vi "Set Position AE.vi"() -> (0 "Cursor Y":dbl)   [LabVIEW 2014]
uses:
  FPGA-7842R-Reference.ctl
panel:
  in  "Set Position":bool
  out "Channel 1":sgl[][](graph)
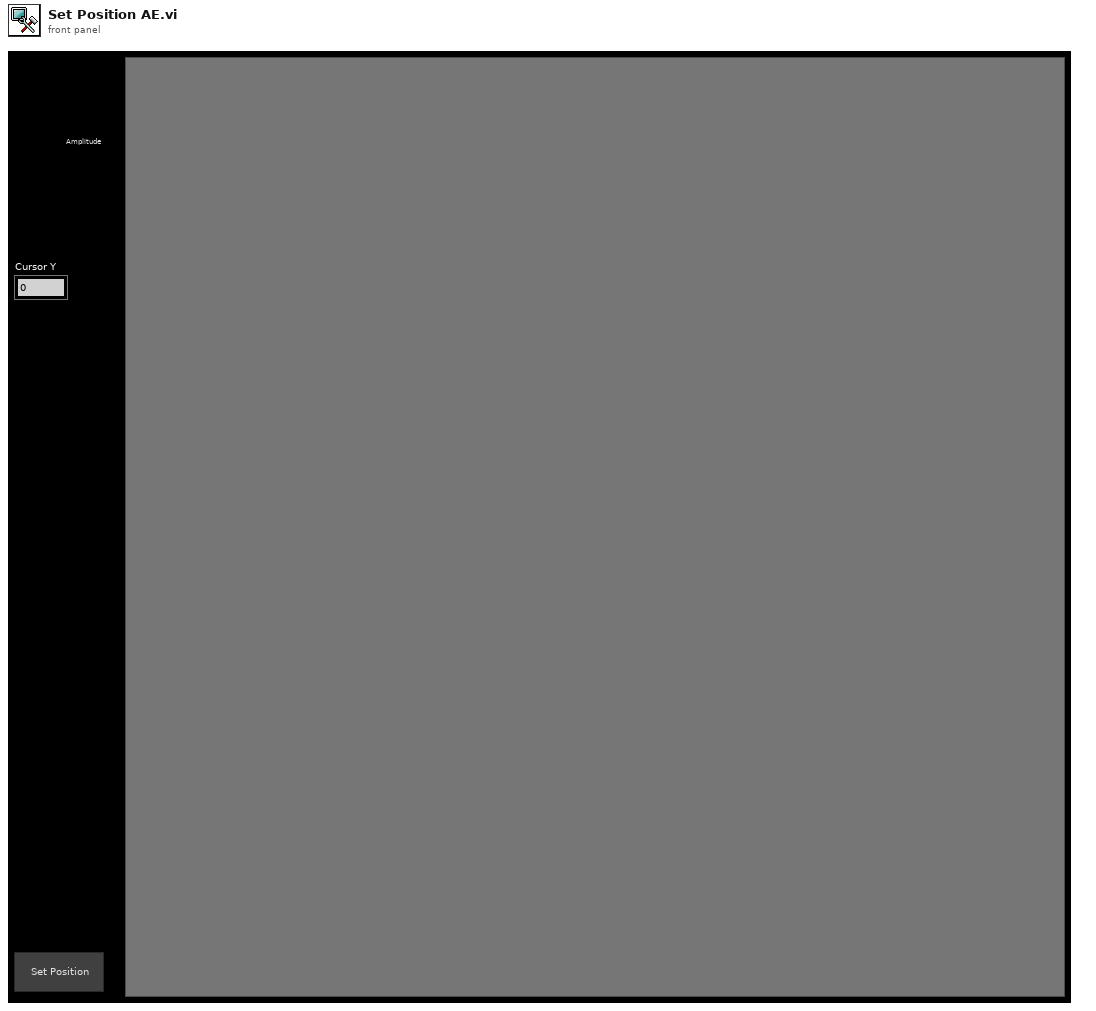
[diagram p1: front panel]
types:
  T1 = typedef "FPGA-7842R-Reference.ctl" = enum16{"Stage Control", "Laser Control", "Unused Axis I16", "Exit", "Set Res Mirror", "Set Galvo", "Current Frame for Capture", "Default", "Close FPGA", "Stop Waveforms", "Start Waveforms", "Shutter Control", "Initialize"}
  T2 = typedef "Image Acquisition Parameters.ctl" = cluster{"Scan Type":enum16{"Sample Scanning", "Beam Scanning"}, "Scan Mode":enum16{"XY", "XZ", "YZ", "XYZ"}, "Fast Axis Frequency (Hz)":dbl, "Image Format":u16, "Line Accumulations":u16, "Frames Per Capture":u16, "Frames Accumulations":u16, "Image Dimension (um)":dbl[], "Number of Z Steps":u16, "Z Steps Size (um)":dbl, "Pixel Size (nm)":dbl[], "Customized Image Format":dbl[]}
  T3 = typedef "Manual Controls V2.ctl" = cluster{"Galvo 1 Position (I16)":i16, "Galvo 2 Position (I16)":i16, "X Axis Voltage (I16)":i16, "Y Axis Voltage (I16)":i16, "Z Axis Voltage (I16)":i16, "Res Mirror Amp (I16)":i16, "Res Mirror Mute":bool, "Upper Shutter":bool, "Lower Shutter":bool}
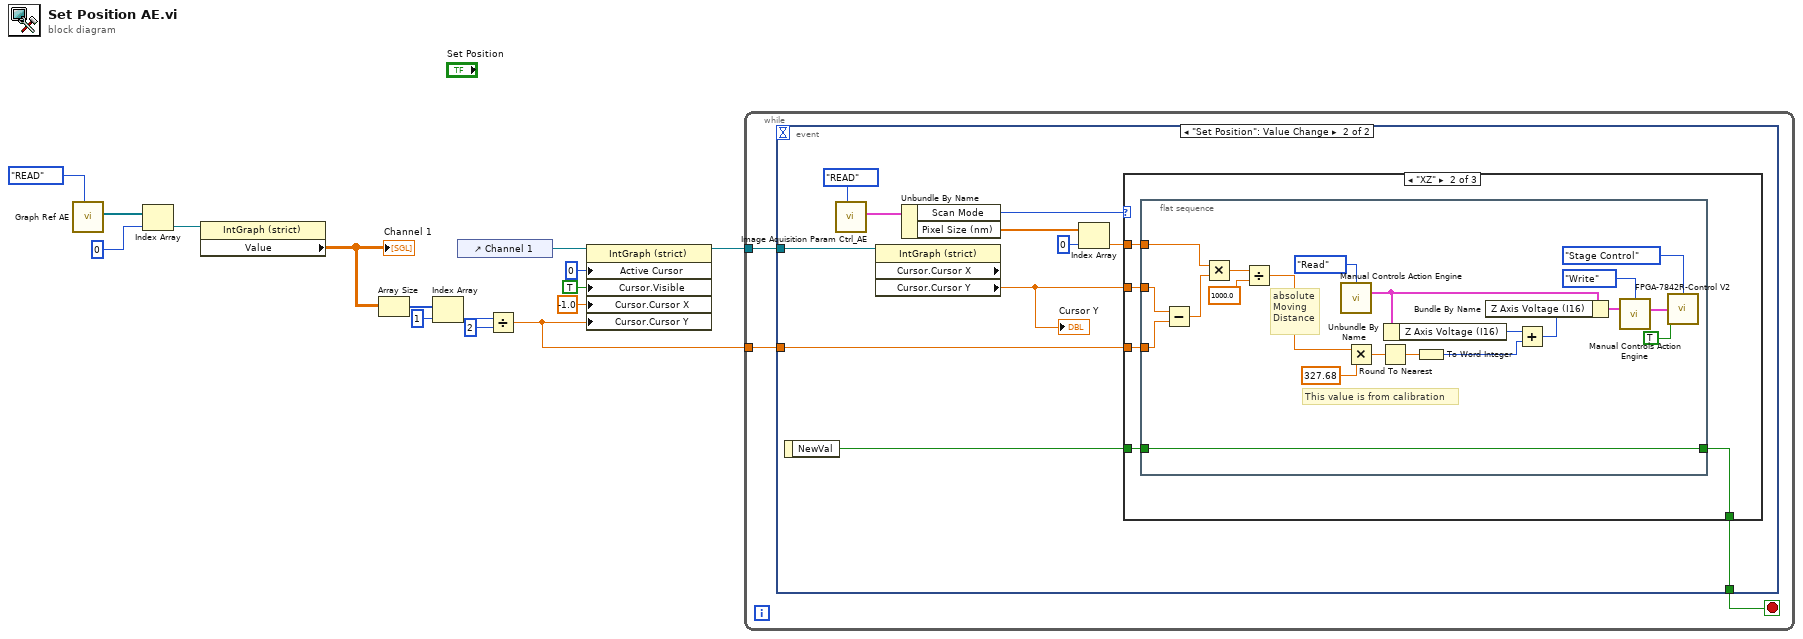
[diagram p0: block diagram]
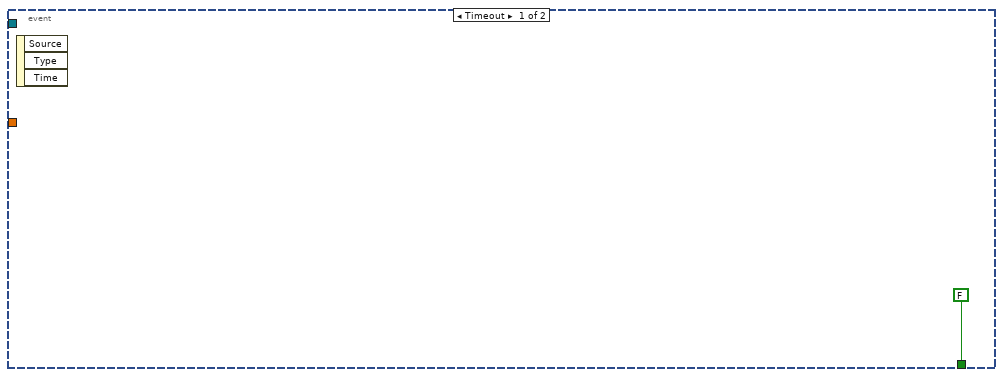
[diagram p2: hidden frame]
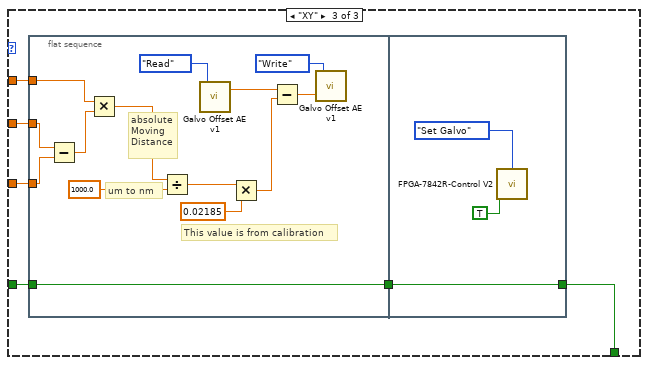
[diagram p4: hidden frame]
diagram:
  n1 = call "Graph Ref AE.vi"("Action"=enum16{"READ", "WRITE"}."READ") -> ("Graph Ref Out"=w11:refnum<vi>[])  [unwired: 10 in]
  n2 = Index Array(array=w11, index=0) -> (element=w9:refnum<vi>)
  n3 = property class="IntGraph (strict)"(reference=w9) -> ("Value"=w4:sgl[][])  [unwired: 1 in, 2 out]
  "Channel 1" <- w4
  n4 = Array Size(array=w4) -> (size(s)=w8:i32[])
  n5 = Index Array(array=w8, index=1) -> (element=w6:i32)
  n6 = control-ref of="Channel 1"() -> (w13:refnum<vi>)
  n7 = Divide(x=w6, y=2) -> (x/y=w1:dbl)
  n8 = property class="IntGraph (strict)"(reference=w13, "Active Cursor"=u32 0, "Cursor.Visible"=TRUE, "Cursor.Cursor X"=-1.0 ("Cursor.Cursor Position:Cursor X"), "Cursor.Cursor Y"=w1) -> (reference out=w2:refnum<vi>)  [unwired: 1 in, 1 out]
  n9 = while {
    tunnel: w2 -> [w18]
    tunnel: w1 -> [w16]
    stop <- w17 stop-if-true
    n10 = event shown="[1] \"Set Position\": Value Change" {
      selector: _ -> [_ _]
      dyn-events: _ -> [_ _]
      timeout: _ -> [_ _]
      tunnel: w18 -> [_ w28]
      tunnel: [FALSE ("NewVal") w21] -> w17
      tunnel: w16 -> [_ w23]
      event Timeout {
        n11 = event-data() -> ()  [unwired: 1 in, 3 out]
      }
      event "Set Position": Value Change {
        n12 = event-data() -> ("NewVal"=w22:bool)  [unwired: 1 in]
        n13 = call "Image Aquisition Param Ctrl_AE.vi"("Action"=enum16{"READ", "WRITE"}."READ") -> ("Image Acquisition Parameters Out"=w30:T2)  [unwired: 10 in]
        n14 = property class="IntGraph (strict)" props=["Cursor", "Cursor X", "Cursor", "Cursor Y"](reference=w28) -> ("Cursor.Cursor Y"=w20:dbl)  [unwired: 1 in, 3 out]
        "Cursor Y" <- w20
        n15 = Unbundle By Name(w30) -> ("Scan Mode"=w29:enum16{"XY", "XZ", "YZ", "XYZ"}, "Pixel Size (nm)"=w26:dbl[])
        n16 = Index Array(array=w26, index=0) -> (element=w24:dbl)
        n17 = case shown="\"XZ\"" w29 {
          tunnel: w24 -> [_ w34 w61]
          tunnel: w20 -> [_ w36 w63]
          tunnel: w23 -> [_ w35 w62]
          tunnel: w22 -> [w31 w33 w59]
          tunnel: [w31 w32 w58] -> w21
          frame Default {
          }
          frame "XZ" {
            n18 = flat-sequence {
              tunnel: w36 -> [w57]
              tunnel: w35 -> [w56]
              tunnel: w34 -> [w54]
              tunnel: [w37] -> w32
              tunnel: w33 -> [w37]
              frame #0 {
                # "This value is from calibration"
                # "absolute\nMoving\nDistance"
                n19 = Subtract(x=w57, y=w56) -> (x-y=w55:dbl)
                n20 = Multiply(x=w54, y=w55) -> (x*y=w53:dbl)
                n21 = Divide(x=w53, y=1000.0) -> (x/y=w38:dbl)
                n22 = call "Manual Controls Action Engine.vi"("Action"=enum16{"Read", "Write"}."Read") -> ("Manual Controls Out"=w46:T3)  [unwired: 14 in]
                n23 = Multiply(x=w38, y=327.68) -> (x*y=w40:dbl)
                n24 = Round To Nearest(number=w40) -> (nearest integer value=w41:dbl)
                n25 = Unbundle By Name(w46) -> ("Z Axis Voltage (I16)"=w43:i16)
                n26 = To Word Integer(number=w41) -> (16bit integer=w44:i16)
                n27 = Add(x=w43, y=w44) -> (x+y=w45:i16)
                n28 = Bundle By Name(cluster=w46, "Z Axis Voltage (I16)"=w45) -> (w47:T3)
                n29 = call "Manual Controls Action Engine.vi"("Action"=enum16{"Read", "Write"}."Write", "Manual Controls In"=w47) -> ("Manual Controls Out"=w49:T3)  [unwired: 13 in]
                n30 = call "FPGA-7842R-Control V2.vi"("Action"=FPGA-7842R-Reference."Stage Control", "Manual Controls"=w49, "Initialize"=TRUE) -> ()  [unwired: 11 in, 2 out]
              }
            }
          }
          frame "XY" {
            n31 = flat-sequence {
              tunnel: w63 -> [w77]
              tunnel: w62 -> [w76]
              tunnel: w61 -> [w74]
              tunnel: [w67] -> w60
              tunnel: w59 -> [w67]
              tunnel: [w78] -> w58
              tunnel: w60 -> [w78]
              frame #0 {
                # "um to nm"
                # "This value is from calibration"
                # "absolute\nMoving\nDistance"
                n32 = Subtract(x=w77, y=w76) -> (x-y=w75:dbl)
                n33 = Multiply(x=w74, y=w75) -> (x*y=w65:dbl)
                n34 = Divide(x=w65, y=1000.0) -> (x/y=w66:dbl)
                n35 = call "Galvo Offset AE v1.vi"("Action"=enum16{"Read", "Write"}."Read") -> ("Galvo 1 Offset Out"=w71:dbl)  [unwired: 1 in, 1 out]
                n36 = Multiply(x=w66, y=0.02185) -> (x*y=w70:dbl)
                n37 = Subtract(x=w71, y=w70) -> (x-y=w69:dbl)
                n38 = call "Galvo Offset AE v1.vi"("Galvo 1 Offset In"=w69, "Action"=enum16{"Read", "Write"}."Write") -> ()  [unwired: 2 out]
              }
              frame #1 {
                n39 = call "FPGA-7842R-Control V2.vi"("Action"=FPGA-7842R-Reference."Set Galvo", "Initialize"=TRUE) -> ()  [unwired: 12 in, 2 out]
              }
            }
          }
        }
      }
    }
  }
